vi "Experiment Dequeuer.vi"(0 "Experiment Queue":refnum<queue>) -> ()   [LabVIEW 2013]
doc: "Run forever, dequeuing items from the given experimental queue and executing the experiments described by those items. This VI fires an event to the occurance in the experimental queue bundle after the experiment has finished."
uses:
  Experimental Configuration.ctl
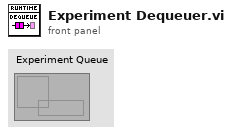
[diagram p1: front panel]
types:
  T1 = typedef "Experimental Configuration.ctl" = cluster{"Output Waveforms":waveform(dbl)[], "Output Channels":string, "Input Channels":string, "Post-Hook Occurence":refnum<k4>}
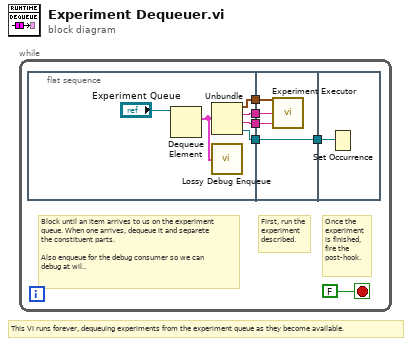
[diagram p0: block diagram]
diagram:
  # "This VI runs forever, dequeuing experiments from the experiment queue as they become available."
  n1 = while {
    stop <- FALSE stop-if-true
    # "Once the\nexperiment\nis finished,\nfire the\npost-hook."
    # "First, run the\nexperiment\ndescribed."
    # "Block until an item arrives to us on the experiment\nqueue. When one arrives, dequeue it and separete\nthe constituent parts.\n\nAlso enqueue for the debug consumer so we can\ndebug at wil.."
    n2 = flat-sequence {
      tunnel: [w11] -> w6
      tunnel: [w10] -> w5
      tunnel: [w9] -> w4
      tunnel: [w8] -> w3
      tunnel: w6 -> [w16]
      tunnel: w5 -> [w15]
      tunnel: w4 -> [w14]
      tunnel: w3 -> [w13]
      tunnel: [w13] -> w2
      tunnel: w2 -> [w17]
      frame #0 {
        n3 = Dequeue Element(queue="Experiment Queue") -> (element=w7:T1)  [unwired: 2 in, 3 out]
        n4 = Unbundle(w7) -> ("Output Waveforms"=w11:waveform(dbl)[], "Output Channels"=w10:string, "Input Channels"=w9:string, "Post-Hook Occurence"=w8:refnum<k4>)
        n5 = call "Lossy Debug Enqueue.vi"("Experimental Configuration"=w7) -> ()
      }
      frame #1 {
        n6 = call "Experiment Executor.vi"("Input Channels"=w14, "Output Channels"=w15, "Output Waveforms"=w16) -> ()
      }
      frame #2 {
        n7 = Set Occurrence(w17) -> ()
      }
    }
  }
